vi "Linear, Exp, and Power Fit.vi"() -> ()   [LabVIEW 2014]
doc: "This example generates data sets and then uses either a linear, exponential, or power fit function to create a best fit line for the data."
uses:
  <vilib>/Analysis/NI_AALPro.lvlib
panel:
  in  "Tab Control":T1(tab)
  in  "method":u16(ring) items=["Least Square", "Least Absolute Residual", "Bisquare"]
  out "residue":dbl format="%#.6g"
  in  "intercept":dbl
  out "fit intercept":dbl format="%#.6g"
  out "fit slope":dbl format="%#.6g"
  in  "Number of points":i32=50
  in  "noise amplitude":dbl=0.8
  in  "slope":dbl=1.0
  out "Linear Model Graph":dbl[][](graph)
  in  "method":u16(ring)=1 items=["Least Square", "Least Absolute Residual", "Bisquare"]
  out "residue":dbl
  out "fit damping":dbl
  out "fit amplitude":dbl
  in  "Number of points":i32=35
  in  "noise amplitude":dbl=0.4
  in  "damping":dbl=0.1
  in  "amplitude":dbl=1.0
  out "Exponential Model Graph":dbl[][](graph)
  out "residue":dbl
  out "fit offset":dbl=2.0
  out "fit damping":dbl=0.1
  out "fit amplitude":dbl=1.0
  in  "Number of points":i32=35
  in  "noise amplitude":dbl=0.4
  in  "offset":dbl=2.0
  in  "damping":dbl=0.1
  in  "amplitude":dbl=1.0
  out "Exponential + offset Model Graph":dbl[][](graph)
  in  "end":dbl=10.0
  in  "start":dbl=1.0
  in  "tolerance":dbl=0.0001 format="%#_3g"
  in  "power method":u16(ring) items=["Least Square", "Least Absolute Residual", "Bisquare"]
  in  "noise amplitude":dbl=0.3
  out "residue":dbl
  out "fit amplitude":dbl
  out "fit power":dbl
  in  "amplitude":dbl=1.0
  in  "power":dbl=2.0
  out "Power Model Graph":dbl[][](graph)
  in  "Number of points":i32=10
  # "Overview: Use a linear, exponential, or power fit function to create a best fit line for generated data.\nRequirements: LabVIEW Full Development System\nInstructions:\n1. Run the VI.\n2. Enter the parameters (i.e. Number of points, a, b, etc.) for the data points to be generated according to the model.  \n3. Select a different tab and run the VI again to view different types of data sets and their corresponding best fit lines."
  # "y = a*x + b + noise"
  # "y = a*exp(b*x) + noise"
  # "y = a*exp(b*x) + c + noise"
  # "y = a*x^b + noise"
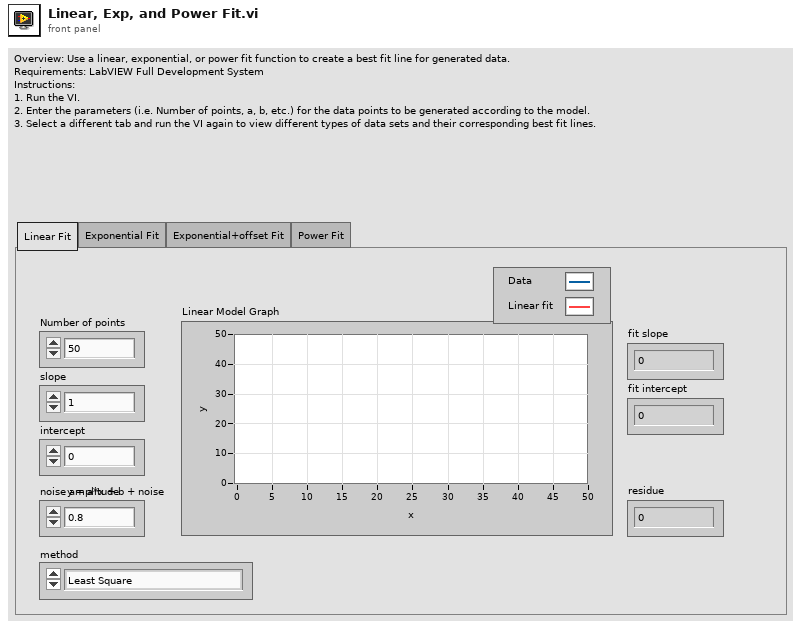
[diagram p1: front panel]
types:
  T1 = enum32{"Linear Fit", "Exponential Fit", "Exponential+offset Fit", "Power Fit"}
  T2 = cluster{"amp min":dbl, "amp max":dbl, "damping min":dbl, "damping max":dbl, "offset min":dbl, "offset max":dbl}
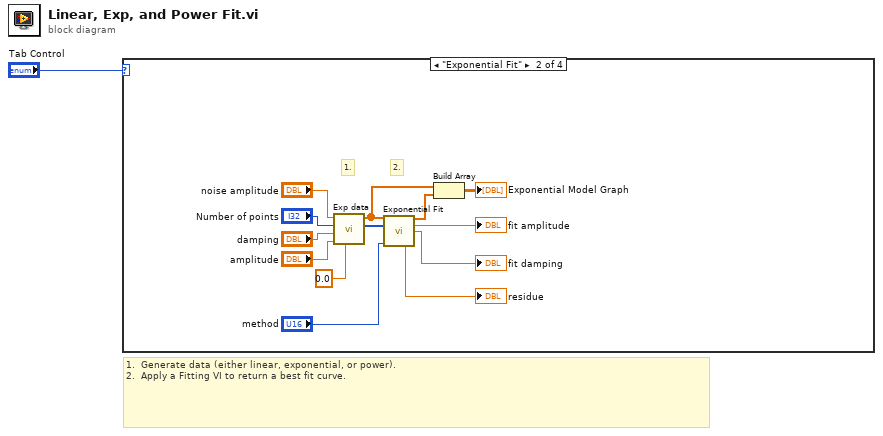
[diagram p0: block diagram]
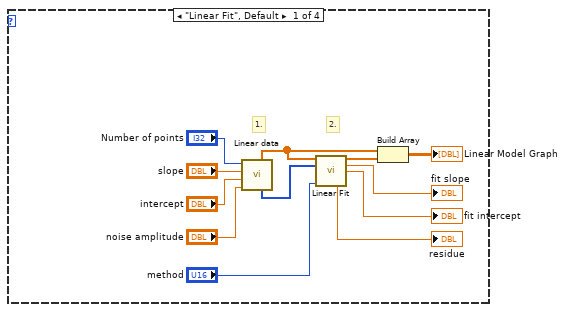
[diagram p2: hidden frame]
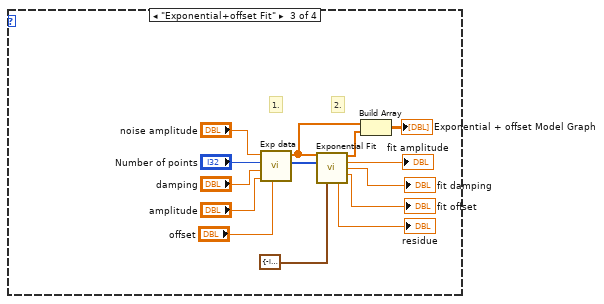
[diagram p3: hidden frame]
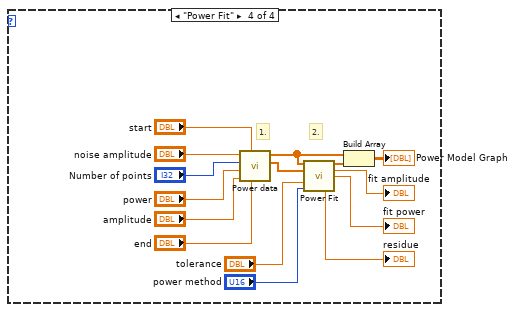
[diagram p4: hidden frame]
diagram:
  # "1.  Generate data (either linear, exponential, or power).\n2.  Apply a Fitting VI to return a best fit curve."
  n1 = case shown="\"Exponential Fit\"" "Tab Control" {
    frame "Linear Fit", Default {
      # "2."
      # "1."
      n2 = call "Linear data.vi"("noise amplitude"="noise amplitude", "b"="intercept", "a"="slope", "Number of points"="Number of points") -> ("X Array"=w10:i32[], "Y Array"=w7:dbl[])  [unwired: 6 in]
      n3 = call <vilib>:"Linear Fit.vi"("Y"=w7, "X"=w10, "method"="method") -> ("Best Linear Fit"=w8:dbl[], "slope"=→"fit slope":dbl, "intercept"=→"fit intercept":dbl, "residue"=→"residue":dbl)  [unwired: 8 in, 1 out]
      n4 = Build Array(w7, w8) -> (→"Linear Model Graph":dbl[][])
    }
    frame "Exponential Fit" {
      # "2."
      # "1."
      n5 = call "Exp data.vi"("c"=0.0, "a"="amplitude", "b"="damping", "Number of points"="Number of points", "noise amplitude"="noise amplitude") -> ("X Array"=w14:i32[], "Y Array"=w15:dbl[])  [unwired: 5 in]
      n6 = call <vilib>:"Exponential Fit.vi"("Y"=w15, "X"=w14, "method"="method") -> ("Best Exponential Fit"=w21:dbl[], "amplitude"=→"fit amplitude":dbl, "damping"=→"fit damping":dbl, "residue"=→"residue":dbl)  [unwired: 7 in, 2 out]
      n7 = Build Array(w15, w21) -> (→"Exponential Model Graph":dbl[][])
    }
    frame "Exponential+offset Fit" {
      # "2."
      # "1."
      n8 = call "Exp data.vi"("c"="offset", "a"="amplitude", "b"="damping", "Number of points"="Number of points", "noise amplitude"="noise amplitude") -> ("X Array"=w32:i32[], "Y Array"=w33:dbl[])  [unwired: 5 in]
      n9 = call <vilib>:"Exponential Fit.vi"("Y"=w33, "X"=w32, "parameter bounds"=T2 {"amp min"=-inf, "amp max"=inf, "damping min"=-inf, "damping max"=inf, "offset min"=-inf, "offset max"=inf}) -> ("Best Exponential Fit"=w31:dbl[], "amplitude"=→"fit amplitude":dbl, "damping"=→"fit damping":dbl, "offset"=→"fit offset":dbl, "residue"=→"residue":dbl)  [unwired: 7 in, 1 out]
      n10 = Build Array(w33, w31) -> (→"Exponential + offset Model Graph":dbl[][])
    }
    frame "Power Fit" {
      # "2."
      # "1."
      n11 = call "Power data.vi"("end"="end", "start"="start", "a"="amplitude", "b"="power", "Number of points"="Number of points", "noise"="noise amplitude") -> ("X Array"=w45:dbl[], "Y Array"=w51:dbl[])  [unwired: 4 in]
      n12 = call <vilib>:"Power Fit.vi"("Y"=w51, "X"=w45, "tolerance"="tolerance", "method"="power method") -> ("Best Power Fit"=w54:dbl[], "amplitude"=→"fit amplitude":dbl, "power"=→"fit power":dbl, "residue"=→"residue":dbl)  [unwired: 6 in, 2 out]
      n13 = Build Array(w51, w54) -> (→"Power Model Graph":dbl[][])
    }
  }
